vi "Demo_Format_String.vi"() -> ()   [LabVIEW 2020]
panel:
  out "Formatted string":string
  in  "Mark":dbl format="%#_13g"
  in  "ID":i32
  in  "User Name":string
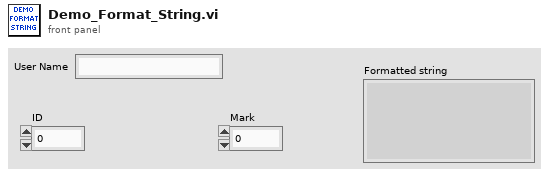
[diagram p1: front panel]
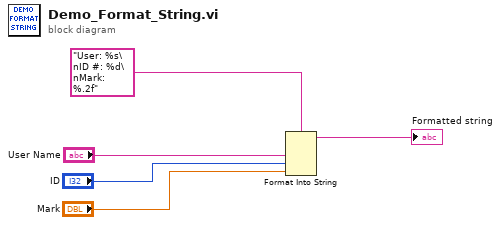
[diagram p0: block diagram]
diagram:
  n1 = Format Into String(format string="User: %s\nID #: %d\nMark: %.2f", "User Name", "ID", "Mark") -> (resulting string=→"Formatted string":string)  [unwired: 2 in, 1 out]
